vi "BB_Image_Process.vi"(9 "LED Color":T2={"Hue"={107.81818389892578, 139.81818389892578}, "Sat"={176.07142857142858, 255.0}, "Val"={40.53571428571429, 255.0}} {"Hue" scale=0.0..255.0 scale format="%#_3g"}, 10 "Mask":T1, 11 "Input Image":T1) -> (2 "Mask":T1(plugin-control), 3 "Original Image":T1(plugin-control))   [LabVIEW 2016]
uses:
  Program Files (x86)/National Instruments/LabVIEW 2016/examples/FRC/roboRIO/Vision/2017 Vision Example/Vision Support Code/Camera Types.ctl
  <vilib>/vision/Image Controls.llb/IMAQ Image.ctl
  <vilib>/vision/NI_Vision_Development_Module.lvlib
panel:
  out "Qualified Particles":i32
  in  "Annotate":bool=TRUE
  out "Results":T3 {"Score" format="%#_3g"; "Pixels"."Rectangle"."Numeric 5" format="%#_3g"; "Pixels"."Rectangle"."Numeric 3" format="%#_3g"; "Pixels"."Rectangle"."Numeric 2" format="%#_3g"; "Pixels"."Rectangle"."Numeric" format="%#_3g"; "Normalized"."Rectangle"."Numeric 5" format="%#_2g"; "Normalized"."Rectangle"."Numeric 3" format="%#_2g"; "Normalized"."Rectangle"."Numeric 2" format="%#_2g"; "Normalized"."Rectangle"."Numeric" format="%#_2g"; "Normalized"."Center"."?" format="%#_3g"; "Normalized"."Center"."?" format="%#_3g"; "Distance (ft)" format="%#_3g"}
  in  "Camera Type":T4=enum."MS HD3000 square"
  in  "Std Devs for Calibration":cluster{"H":dbl, "S":dbl, "V":dbl}={"H"=4.0, "S"=6.0, "V"=6.0}
  in  "Score Cutoff %":dbl=70.0
  in  "Particles":dbl=5.0
  in  "Color Mode":u16(ring)=3 items=["RGB", "HSL", "HSV", "HSI"]
  in  "Use Calibration":bool=TRUE
  in  "Line Border":cluster{"Top":dbl, "Bottom":dbl}={"Top"=6.0, "Bottom"=1.0}
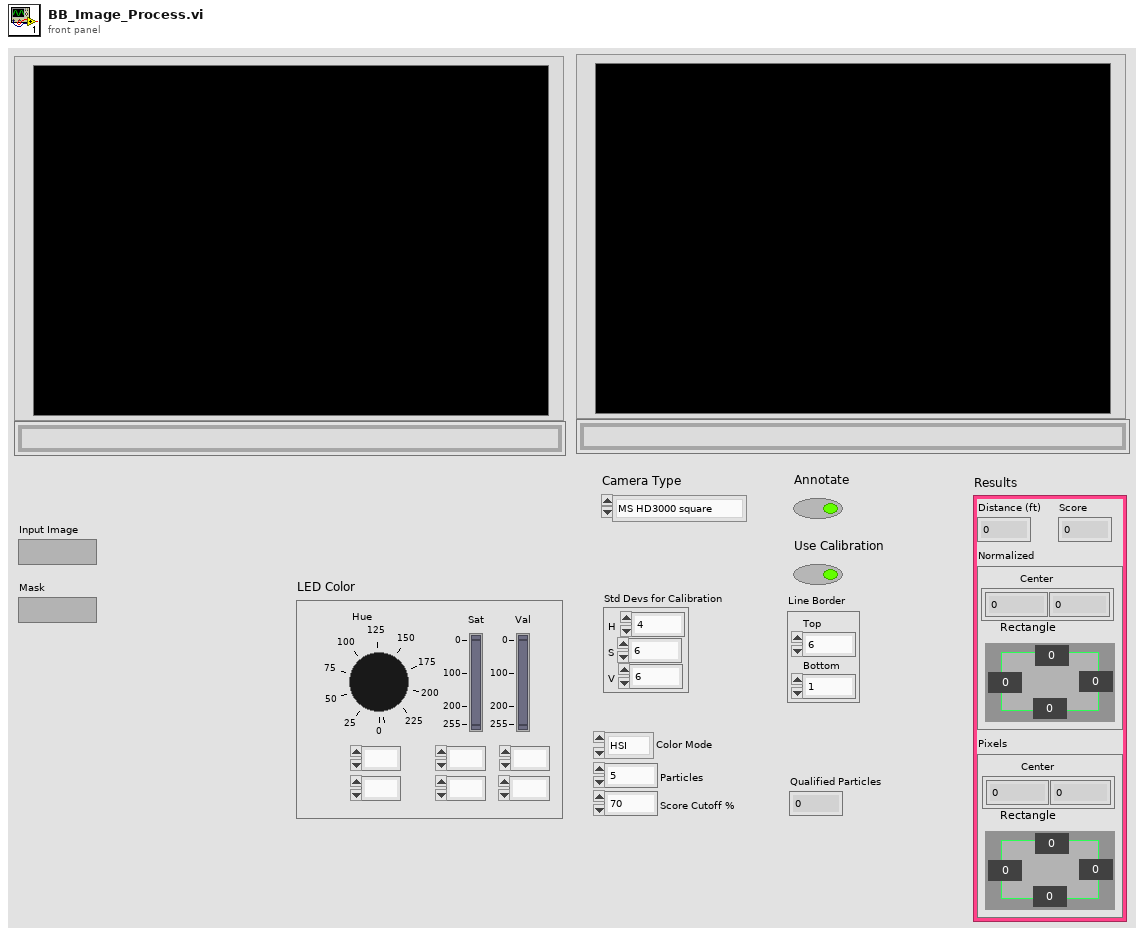
[diagram p1: front panel]
types:
  T1 = typedef "IMAQ Image.ctl" = refnum<image>
  T2 = cluster{"Hue":cluster{dbl, dbl}, "Sat":cluster{dbl, dbl}, "Val":cluster{dbl, dbl}}
  T3 = cluster{"Distance (ft)":dbl, "Score":dbl, "Normalized":cluster{"Center":cluster{dbl, dbl}, "Rectangle":cluster{"Numeric":dbl, "Numeric 2":dbl, "Numeric 3":dbl, "Numeric 5":dbl}}, "Pixels":cluster{"Center":cluster{dbl, dbl}, "Rectangle":cluster{"Numeric":dbl, "Numeric 2":dbl, "Numeric 3":dbl, "Numeric 5":dbl}}}
  T4 = typedef "Camera Types.ctl" = enum16{"206", "1011", "1013", "MS HD3000 square", "MS HD3000 640x480"}
  T5 = typedef "Image Type" = u32
  T6 = typedef "Particle Parameters" = i32
  T7 = cluster{cluster{dbl, dbl}, cluster{dbl, dbl}, cluster{dbl, dbl}}
  T8 = cluster{"Left":dbl, "Top":dbl, "Right":dbl, "Bottom":dbl}
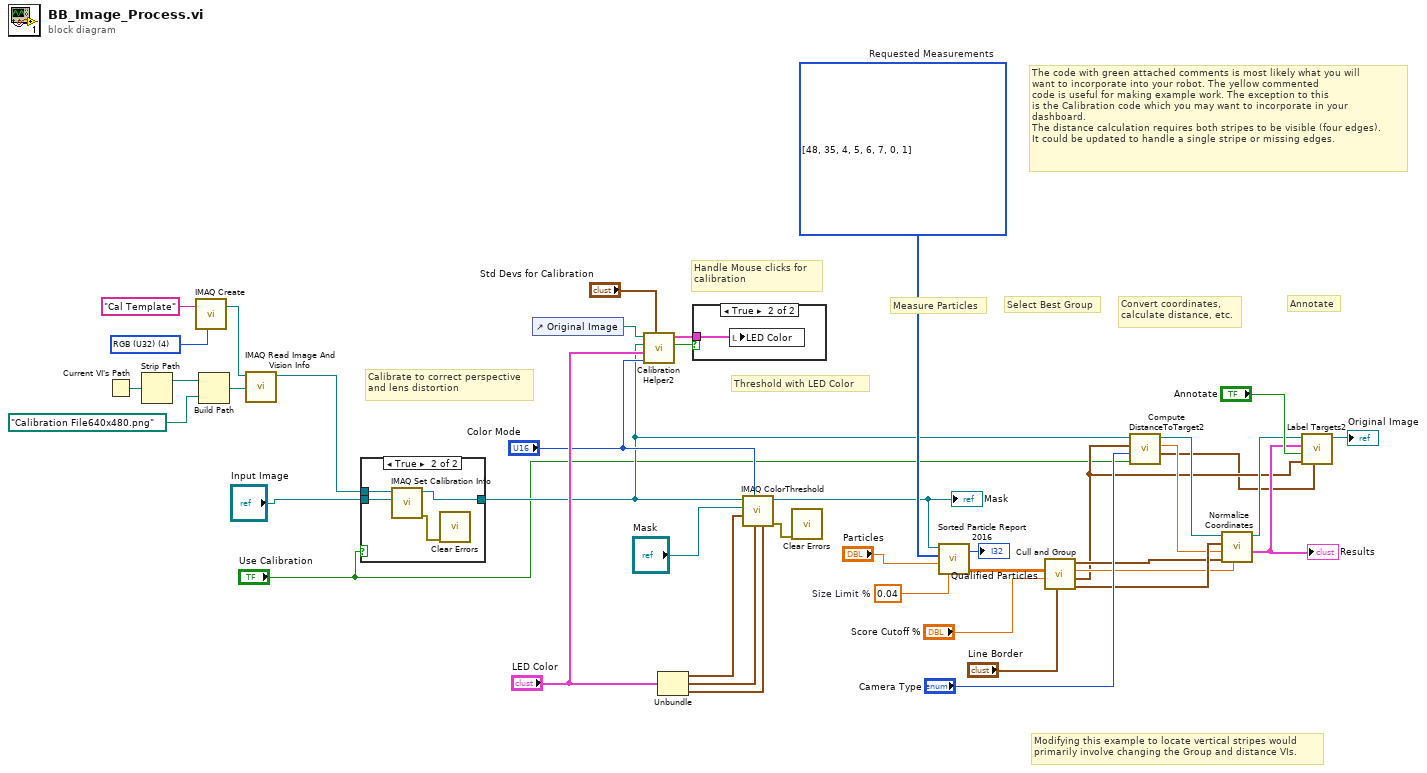
[diagram p0: block diagram]
diagram:
  w29 = 0.04  # Size Limit %
  w41 = T5 4 items=["Grayscale (U8)", "Grayscale (I16)", "Grayscale (SGL)", "Complex (CSG)", "RGB (U32)", "HSL (U32)", "RGB (U64)", "Grayscale (U16)"] ("Image Type")
  w42 = T6[] [48, 35, 4, 5, 6, 7, 0, 1] items=["Center of Mass X", "Center of Mass Y", "First Pixel X", "First Pixel Y", "Bounding Rect Left", "Bounding Rect Top", "Bounding Rect Right", "Bounding Rect Bottom", "Max Feret Diameter Start X", "Max Feret Diameter Start Y", "Max Feret Diameter End X", "Max Feret Diameter End Y", "Max Horiz. Segment Length Left", "Max Horiz. Segment Length Right", "Max Horiz. Segment Length Row", "-", "Bounding Rect Width", "Bounding Rect Height", "Bounding Rect Diagonal", "Perimeter", "Convex Hull Perimeter", "Holes' Perimeter", "Max Feret Diameter", "Equivalent Ellipse Major Axis", "Equivalent Ellipse Minor Axis", "Equivalent Ellipse Minor Axis (Feret)", "Equivalent Rect Long Side", "Equivalent Rect Short Side", "Equivalent Rect Diagonal", "Equivalent Rect Short Side (Feret)", "Average Horiz. Segment Length", "Average Vert. Segment Length", "Hydraulic Radius", "Waddel Disk Diameter", "-", "Area", "Holes' Area", "Particle & Holes' Area", "Convex Hull Area", "Image Area", "-", "Number of Holes", "Number of Horiz. Segments", "Number of Vert. Segments", "-", "Orientation", "Max Feret Diameter Orientation", "-", "% Area/Image Area", "% Area/(Particle & Holes' Area)", "Ratio of Equivalent Ellipse Axes", "Ratio of Equivalent Rect Sides", "-", "Elongation Factor", "Compactness Factor", "Heywood Circularity Factor", "Type Factor", "-", "Sum X", "Sum Y", "Sum XX", "Sum XY", "Sum YY", "Sum XXX", "Sum XXY", "Sum XYY", "Sum YYY", "-", "Moment of Inertia XX", "Moment of Inertia XY", "Moment of Inertia YY", "Moment of Inertia XXX", "Moment of Inertia XXY", "Moment of Inertia XYY", "Moment of Inertia YYY", "Norm. Moment of Inertia XX", "Norm. Moment of Inertia XY", "Norm. Moment of Inertia YY", "Norm. Moment of Inertia XXX", "Norm. Moment of Inertia XXY", "Norm. Moment of Inertia XYY", "Norm. Moment of Inertia YYY", "Hu Moment 1", "Hu Moment 2", "Hu Moment 3", "Hu Moment 4", "Hu Moment 5", "Hu Moment 6", "Hu Moment 7"]  # Requested Measurements
  # "Calibrate to correct perspective\nand lens distortion"
  # "Handle Mouse clicks for\ncalibration"
  # "Measure Particles"
  # "Convert coordinates,\ncalculate distance, etc."
  # "Annotate"
  # "Select Best Group"
  # "Threshold with LED Color"
  # "Modifying this example to locate vertical stripes would\nprimarily involve changing the Group and distance VIs."
  # "The code with green attached comments is most likely what you will\nwant to incorporate into your robot. The yellow commented\ncode is useful for making example work. The exception to this\nis the Calibration code which you may want to incorporate in your\ndashboard.\nThe distance calculation requires both stripes to be visible (four edges).\nIt could be updated to handle a single stripe or missing edges."
  n1 = Current VI's Path() -> (path=w37:path)
  n2 = Strip Path(path=w37) -> (stripped path=w34:path)  [unwired: 1 out]
  n3 = call "IMAQ Create"("Image Name"="Cal Template", "Image Type"=w41) -> ("New Image"=w39:T1)  [unwired: 2 in, 2 out]
  n4 = Build Path(base path=w34, name or relative path=path "Calibration File640x480.png" ("Folder Location")) -> (appended path=w36:path)
  n5 = call "IMAQ Read Image And Vision Info"("File Path"=w36, "Image"=w39) -> ("Image Out"=w38:T1)  [unwired: 7 in, 2 out]
  n6 = case shown="True" "Use Calibration" {
    tunnel: [w43 w47] -> w5
    tunnel: "Input Image" -> [w43 w44]
    tunnel: w38 -> [_ w46]
    frame False {
    }
    frame True {
      n7 = call "IMAQ Set Calibration Info"("Image Dst"=w44, "Image Src"=w46) -> ("error out"=w45:errorcluster, "Calibrated Image"=w47:T1)  [unwired: 8 in]
      n8 = call <vilib>:"Clear Errors.vi"("error in (no error)"=w45) -> ()  [unwired: 5 in, 2 out]
    }
  }
  n9 = control-ref of="Original Image"() -> (w25:refnum<vi>)
  n10 = call "Calibration Helper2.vi"("Std Devs"="Std Devs for Calibration", "Color Mode"="Color Mode", "Color Components"="LED Color", "Image"=w5, "Image Ctl Refnum"=w25) -> ("Changed"=w24:bool, "output color"=w23:T7)  [unwired: 5 in]
  n11 = Unbundle("LED Color") -> ("Hue"=w33:cluster{dbl, dbl}, "Sat"=w32:cluster{dbl, dbl}, "Val"=w31:cluster{dbl, dbl})
  n12 = case shown="True" w24 {
    tunnel: w23 -> [_ w48]
    frame False {
    }
    frame True {
      n13 = local write "LED Color"(w48) -> ()
    }
  }
  n14 = call "IMAQ ColorThreshold"("Blue or Luma or Val or Inten Range"=w31, "Green or Sat Range"=w32, "Color Mode"="Color Mode", "Red or Hue Range"=w33, "Image Dst"="Mask", "Image Src"=w5) -> ("error out"=w26:errorcluster, "Image Dst Out"=w18:T1)  [unwired: 4 in]
  "Mask" <- w18
  n15 = call <vilib>:"Clear Errors.vi"("error in (no error)"=w26) -> ()  [unwired: 5 in, 2 out]
  n16 = call "Sorted Particle Report 2016.vi"("Min Area Size %"=w29, "Particle Count Limit"="Particles", "Pixel Measurements"=w42, "Image in"=w18) -> ("Sorted Data"=w20:dbl[][], "Particles"=→"Qualified Particles":i32)
  n17 = call "Cull and Group.vi"("Line Border"="Line Border", "Score Cutoff"="Score Cutoff %", "Sorted Data"=w20) -> ("Rect"=w16:T8, "Line"=w7:T8, "Score"=w10:dbl, "Center"=w12:cluster{"X":dbl, "Y":dbl})  [unwired: 5 in]
  n18 = call "Compute DistanceToTarget2.vi"("Calibrated"="Use Calibration", "Camera Type"="Camera Type", "Line"=w7, "Image Src"=w5) -> ("Edges"=w6:cluster{"X":sgl, "Y":sgl}[], "Distance (ft)"=w15:dbl, "Image Dst Out"=w14:T1)  [unwired: 5 in]
  n19 = call "Normalize Coordinates.vi"("Score"=w10, "Center"=w12, "Distance"=w15, "Bounding box"=w16, "Image in"=w14) -> ("Results"=w11:T3, "Image out"=w13:T1)  [unwired: 5 in]
  "Results" <- w11
  n20 = call "Label Targets2.vi"("Edges"=w6, "Line"=w7, "Annotate"="Annotate", "Results"=w11, "Image in"=w13) -> ("Image out"=→"Original Image":T1)  [unwired: 6 in]
